vi "Process Data.vi"(6 "dt":dbl, 8 "error in (no error)":errorcluster, 9 "t0":dbl, 10 "Data":dbl[][](array[numeric]), 11 "DataLogger in":refnum<class "DataLogger.lvclass">) -> (0 "error out":errorcluster, 2 "Processed Data":dbl[][](array[numeric]), 3 "DataLogger out":refnum<class "DataLogger.lvclass">)   [LabVIEW 2020, in "VolatusDataLogger.lvlib" / "DataLogger.lvclass"]
uses:
  DataLogger.lvclass
  DataLogger.lvclass/DataLogger.ctl
  Volatus/Task/Task.lvclass
  C:/dev/lv20CE/relink/lv-volatus/Volatus/DataHandlerTask/DataHandlerTask.lvclass
  C:/dev/lv20CE/relink/lv-volatus/Volatus/Task/Task.lvclass
  C:/Program Files (x86)/National Instruments/LabVIEW 2020/vi.lib/ActorFramework/Actor/Actor.lvclass
  C:/dev/lv20CE/relink/lv-volatus/Volatus/TaskStateHandler/TaskStateHandler.lvclass
  C:/dev/lv20CE/relink/lv-volatus/Volatus/VectoMessageHandler/VectoMessageHandler.lvclass
  C:/dev/lv20CE/relink/lv-volatus/Volatus/API Provider/API Provider.lvclass
  C:/dev/lv20CE/relink/lv-volatus/Volatus/DataHandler/DataHandler.lvclass
  C:/dev/lv20CE/relink/lv-volatus/VolatusDataLogger/DataLogger/DataLogger.lvclass
  C:/dev/lv20CE/relink/lv-volatus/VolatusDataLogger/LoggingHandler/LoggingHandler.lvclass
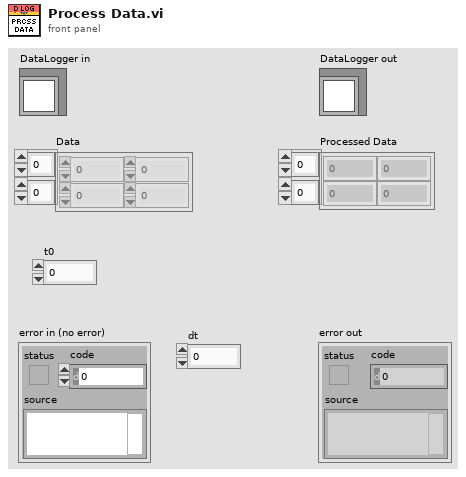
[diagram p1: front panel]
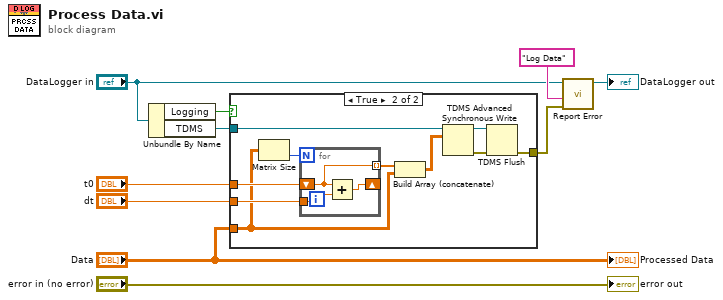
[diagram p0: block diagram]
diagram:
  n1 = Unbundle By Name("DataLogger in") -> ("Logging"=w9:bool, "TDMS"=w8:refnum<k34>)
  n2 = case shown="True" w9 {
    tunnel: "Data" -> [_ w11]
    tunnel: "t0" -> [_ w19]
    tunnel: "dt" -> [_ w18]
    tunnel: w8 -> [_ w16]
    tunnel: [_ w12] -> w7
    frame False {
    }
    frame True {
      n3 = Matrix Size(0:w11) -> (2:w20:i32)  [unwired: 1 out]
      n4 = for {
        N: w20 -> [_]
        tunnel: w18 -> [w23]
        shift-right: [w22] -> _
        shift-left: w19 -> [w21]
        tunnel: [w21] -> w17 mode=indexing
        n5 = Add(x=w21, y=w23) -> (x+y=w22:dbl)
      }
      n6 = Build Array (concatenate)(w17, w11) -> (w15:dbl[][])
      n7 = TDMS Advanced Synchronous Write(10:w15, 11:w16) -> (0:w13:errorcluster, 3:w14:refnum<k34>)  [unwired: 1 in]
      n8 = TDMS Flush(4:w13, 7:w14) -> (0:w12:errorcluster)  [unwired: 1 out]
    }
  }
  n9 = call "Report Error.vi"("error in (no error)"=w7, "Message"="Log Data", "Task in"="DataLogger in") -> ("Task out"=→"DataLogger out":refnum<class "DataLogger.lvclass">)  [unwired: 7 in, 1 out]
  "error out" <- "error in (no error)"
  "Processed Data" <- "Data"
